vi "LabVIEW JSON Example LVJSON Set.vi"() -> ()   [LabVIEW 2019]
uses:
  lib/labview_json.lvlib
panel:
  out "Exists?":bool
  in  "JSON Path":string[](array[string])=["members", "0"]
  in  "JSON to Merge":string="{\"name\":\"MY NEW NAME!\",\n\"age\":999999}"
  in  "JSON in":string="{\n    \"squadName\":\"Super hero squad\",\n    \"homeTown\":\"Metro City\",\n    \"formed\":2016,\n    \"secretBase\":\"Super tower\",\n    \"active\":true,\n    \"members\":[\n        {\n            \"name\":\"Molecule Man\",\n            \"age\":29,\n            \"secretIdentity\":\"Dan Jukes\",\n            \"powers\":[\n                \"Radiation resistance\",\n                \"Turning tiny\",\n                \"Radiation blast\"\n            ]\n        },\n        {\n            \"name\":\"Madame Uppercut\",\n            \"age\":39,\n            \"secretIdentity\":\"Jane Wilson\",\n            \"powers\":[\n                \"Million tonne punch\",\n                \"Damage resistance\",\n                \"Superhuman reflexes\"\n            ]\n        },\n        {\n            \"name\":\"Eternal Flame\",\n            \"age\":1000000,\n            \"secretIdentity\":\"Unknown\",\n            \"powers\":[\n                \"Immortality\",\n                \"Heat Immunity\",\n                \"Inferno\",\n                \"Teleportation\",\n                \"Interdimensional travel\"\n            ]\n        }\n    ]\n}"
  out "error out 3":errorcluster
  out "JSON out":string
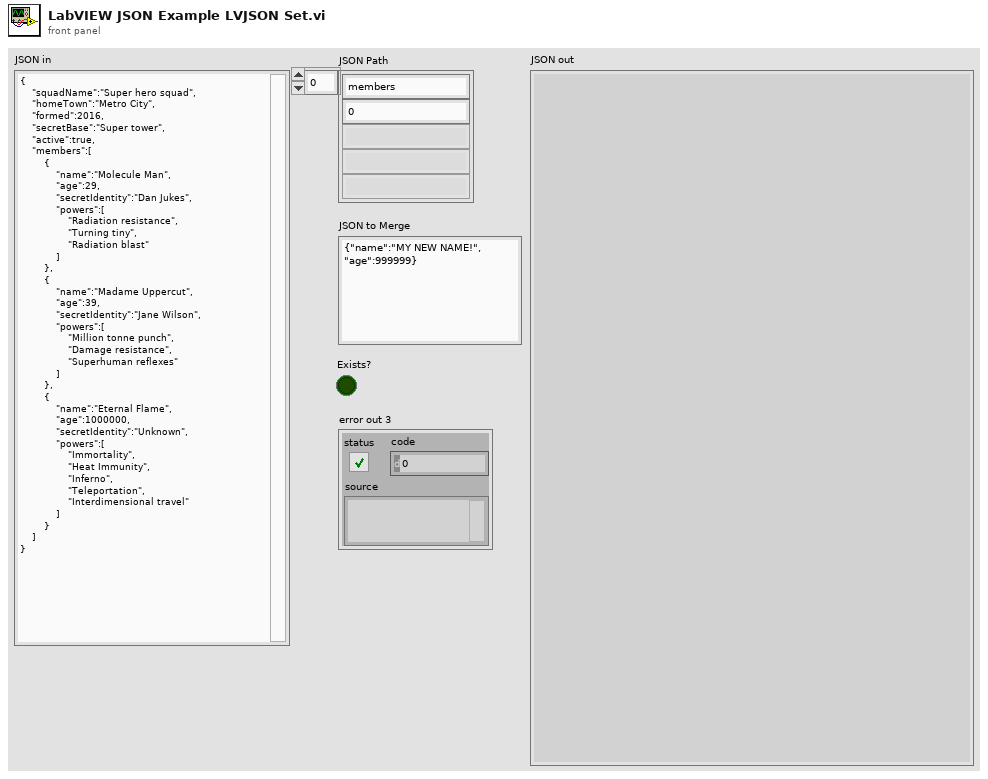
[diagram p1: front panel]
types:
  T1 = typedef "labview_json.lvlib/Element.ctl" = cluster{"Key":string, "Type":T2, "Value":variant}
  T2 = typedef "labview_json.lvlib/Element Type.ctl" = enum8{"NULL", "OBJECT", "ARRAY", "BOOL", "INT", "UINT", "FLOAT", "STRING"}
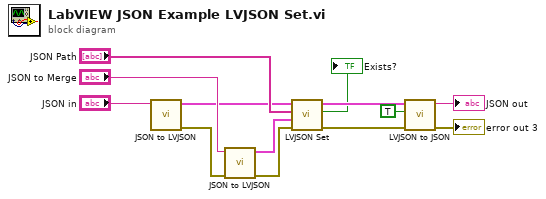
[diagram p0: block diagram]
diagram:
  n1 = call "JSON to LVJSON.vi"("JSON in"="JSON in") -> ("error out"=w1:errorcluster, "Root Element out"=w2:T1)  [unwired: 9 in]
  n2 = call "JSON to LVJSON.vi"("error in (no error)"=w1, "JSON in"="JSON to Merge") -> ("error out"=w5:errorcluster, "Root Element out"=w9:T1)  [unwired: 8 in]
  n3 = call "LVJSON Set.vi"("error in (no error)"=w5, "Element"=w9, "Root Path"="JSON Path", "Root Element in"=w2) -> ("error out"=w12:errorcluster, "Exists?"=→"Exists?":bool, "Root Element out"=w11:T1)  [unwired: 5 in]
  n4 = call "LVJSON to JSON.vi"("error in (no error)"=w12, "Pretty Print? (F)"=TRUE, "Root Element in"=w11) -> ("error out"=→"error out 3":errorcluster, "JSON out"=→"JSON out":string)  [unwired: 6 in, 1 out]
